vi "Main_16b.vi"() -> ()   [LabVIEW 2023]
uses:
  ENUM_Type.ctl
  Cluster_Tracking point.ctl
  Cluster_Point.ctl
  ENUM_Direction_a2.ctl
  Map_Direction Next.ctl
panel:
  out "left":i32
  out "Answer 2":i32
  out "Array 2":cluster{"Track Point":T1[]}[](array[cluster])
  out "Array":T4[][](array[typedef])
  in  "Puzzle":string="\\.......................|..-.............../../.......|...............\\.\\.....|..../.............|............\n........................../....../..............................-............-.-..--.........-...........\\/...\n....\\............../...........-...-......|.............................\\...............-........-....|.......\n......\\....|................./.\\................/..................../.......................|..\\......-......\n.................../..................-./.................../.....-...................|......\\.......|\\...\\./.\n.....|........../....................\\../..\\.../.\\.......-.............\\...........\\......|.\\..-..........-...\n..../............/.....\\...................../..--\\........|......\\....-...|.-...../......-........../........\n..............\\.-............./........./....|\\.......\\..........|.................|.|.................-......\n.....|..........-................-.../..........-........................\\.......|.........................-..\n.|.-......./....................\\........-.............../..\\.|.-\\...........\\./.................-............\n................|/............................../..-.\\..................-..../../...../.../..../..........|...\n........................./.....................\\..\\....-....../-.....................\\|.........././.-........\n...\\.....................-...../|............--......-..|...../.....|......|.../.\\....|.............\\|.......\\\n.........-...-.....|.........../...-/........|......./|............-.......-.....\\.............\\|....../......\n.....|...|.................|...../.............|.................../..........\\|..\\......|..|....-............\n...........................-.........\\......\\.............\\...................-.....-.\\.......-.....|.........\n.................-.............-......./.............-..\\./......|....-..-..........-....-............\\.......\n.\\..\\.......-......|........................\\.............-.......................|.........|\\.|..\\......--/..\n..........-.....||--........|........-....../...........|../...-.........../.....-.\\..........|.......-.......\n..........\\..........|..................\\.................-..../............/..........|.......-........../...\n..--......../..........-..|........./.........-...../........-.................|..\\............../.....-......\n.....\\.............|...../......../............./||..........................\\............|...................\n..-.................-|..-....................\\.................|...\\.....\\............./......-.......\\.......\n............-../......\\...../.-....-.....-....-./../......\\..|..|............................|.../..|.........\n-................./................................................|...............|....|.....-.....|....../..\n...........-...................|...........\\.......-..\\.......-...........|..-....../........|...............|\n.........|...|-........../...-..........|.........\\.....||......./....|...............\\......-......\\...../...\n....|.........|............\\.-.......................................-.......................|.-..|.\\...\\.-...\n.|....|....-/....................\\\\..........................|........\\|...|..............\\..|......-.\\../....\n..|.\\......|..../.....|.......-....................|.\\..\\............/......................|.....\\../../.....\n.......|\\\\.\\/......................./.............|................../.........|.....\\-.......................\n......................................../.../................\\-..............-................./......\\.......\n............../............/\\......./........................./......|............\\/..........................\n......./................|......../.........-............\\.../.|....../....|...../..../......../...............\n...................|............-\\........../...\\.......\\....\\.....-.........-./....|.........................\n.....-..-\\.................|\\...........................|..........\\........-...|.............................\n..............................-.............-.......\\......................../.......\\|.......|...-....-......\n\\...................\\..../.................\\................|......-...-............./.-......................\n........................./.|./...|..\\.-............|.-.....-..........\\....-..../.....|.......|...............\n.................../......../..................|.|...............|.......|\\.....|......|...............\\/..|..\n.........|....-......../........-./..|.../..|./...................-........|..................................\n..|../............-......-.........................-..|....-................-..\\....../...........|...........\n....................-...............|.../.....|..../......../...|.......\\.....-.....\\..............-..\\.-.....\n...........\\.........../............................................\\......-................-.......|.....-...\n..-............./.......-\\...........|-..-../............../................................../...............\n.................\\.......\\............../.|.......-...\\............................................\\.-........\n.\\....|....\\......|........./.....--......................................|................\\..|-..............\n......../...............-..........................|...........................-.............-\\.-..|..........\n.......|......|/...\\........./......../.....\\.........\\.......................-...........\\..\\................\n.-..-../.............|................./../.................\\........-......|.\\.....||...................\\|...\n/......../....\\.....|-..........\\..............-.....|............/\\......\\...//....................\\...-/....\n................-...........-.-\\-..........\\.-./......../-................./../.\\........................./...\n-.........-.....|.....-..|..|.........|...................-..........\\/.-.....................................\n......./...../......\\............-.|...............|..../.........|....\\.................../..............|...\n...........|.......|....|...............\\........................\\/..\\......................................\\.\n......\\........-.........................\\..........\\.............\\......................\\/.....\\..|..........\n......\\...........|.........../..-............./........................../...-......../...............\\..|...\n..|............\\../........../............\\...|.......................-...............\\-../.|...|\\.....\\......\n.|....\\.|....-|.........\\......./.................../.|........|....../.--.\\.....\\..............-\\\\.........-.\n......................./.......\\...........|.\\............-.....\\.............\\.........--......../.\\..-.|../.\n......../.............../......\\.\\....|.............../...........................-........-......../.........\n.......|\\.............|.../|/........../....\\.....-....|.............-......./........\\..\\........\\..|......-.\n.............../...........-.....\\..\\....-...../...|......\\...........................\\...|...........|/......\n.............|....../.................../..|.....................|.......|....//..............\\...............\n......./....\\............................-.........................-/......../|......-....|.............../...\n...........................|...................\\...............................-.................|...........\\\n.............................-......./..../...................\\.../...........-.|......................||.....\n\\....\\....\\...-./......../.........\\................./................\\...................|...........-.......\n................-.../............/\\..................\\.\\..-....../................./..........|...............\n......../...\\.......................\\.......\\..\\......|.....|../..........\\..........-.............|..........\n../.........................................-\\..........-.........|-./.....-...|..|.......\\........-...../../.\n.....|..........-......../|-..............|.................-...........|...\\.....................\\...........\n.......|..............\\....\\.....-............../..\\\\..\\.......-........./.........-..|...|................../\n..........-.......-.-................../.........\\\\...../.....|..........\\......./.|.............-...........\\\n..................................-..................|...........\\../\\...../..../...\\................/........\n...-.........................................................\\.|..............\\..................\\............\n-.|..|...................../../.|.......\\.....|.....\\.\\...\\.........-.................................../.....\n...\\./....../........\\.......-.................\\.........|............-.........../...........\\.|.........|.\\.\n..........-...\\.............-.-............-.-................/.....................|........|............-...\n|......./............/..|..............\\...............|.......|\\................/....|.........|.........\\..\\\n.....\\../\\./.....................-.............\\..................|.|.........................................\n............/......../.../.......\\............/.........................\\........................\\............\n....../..|.............../....................-.......\\................................................|.....\\\n................................../.......././.......\\.....|.\\......-.........-..||......../........-.//......\n........................\\.......|............-....-...../..............................-............-....|...-\n.....-.......|......\\..|.........-....|......\\......../..../.......\\..........|....\\.............||..\\........\n..........|...........-|.......\\.......-....../...../..........||.......................\\............-..|.....\n.................../../..............................|....|................/........|-....|................/..\n.....................\\................/............................/-........./...|.............\\...|..|\\.....\n.....\\..\\..........\\......../......|.........-....-..-..|...........\\....|./....\\.\\..\\............../.........\n.......-...............-....../...........-.......................|../...............|...|.........../..../...\n.............|.../..................\\..\\..........-........||................\\/...........-|..................\n.............-..............-\\.../.................|......\\...../..........\\...-.....-....../................\\\n.....-....................................-.........\\/............../.............................|...........\n./.|../......\\\\..........................................|..............\\|/..-\\..........................\\....\n...........-.........\\............./....-........-....-....-.........\\..\\....-\\...-...............--.........-\n..\\.............................\\............................./\\..........-.............-...-./........../....\n.................../........\\....|..-....|||./..............-......-./....................../..|...|..........\n......\\.........../............|\\...|.-................../....................|\\..|..\\.............-./......|.\n...........-...................-.|........................\\...............|/..-...\\...|/\\...........|.........\n............|..../..................................\\.......................\\........................-........\n.\\..........................|......|......../.|....................../.......\\......\\.............../.........\n..........-.../............/..........................|....-......................|.-................|.-......\n......../............-...|.....|......../-.....-|...|./.......-..................-\\...........................\n...............\\.\\/.-....././................-.../..../.............../-|.....-.......|......./..--...........\n..........-\\\\.|-................./../..|.-.....--................../.................../.|.......-............\n..\\.................-..............-...............\\.....|......................./..\\.....--........./..../..\\\n.......-....../..............|..................\\....|..|..........-.....|.|.-.........................\\......\n..../..\\...\\....................................||.|......................................|.......\\/.........-\n................\\-.-.....||....\\.........................-...................................................|"
  in  "Example":string=".|...\\....\n|.-.\\.....\n.....|-...\n........|.\n..........\n.........\\\n..../.\\\\..\n.-.-/..|..\n.|....-|.\\\n..//.|...."
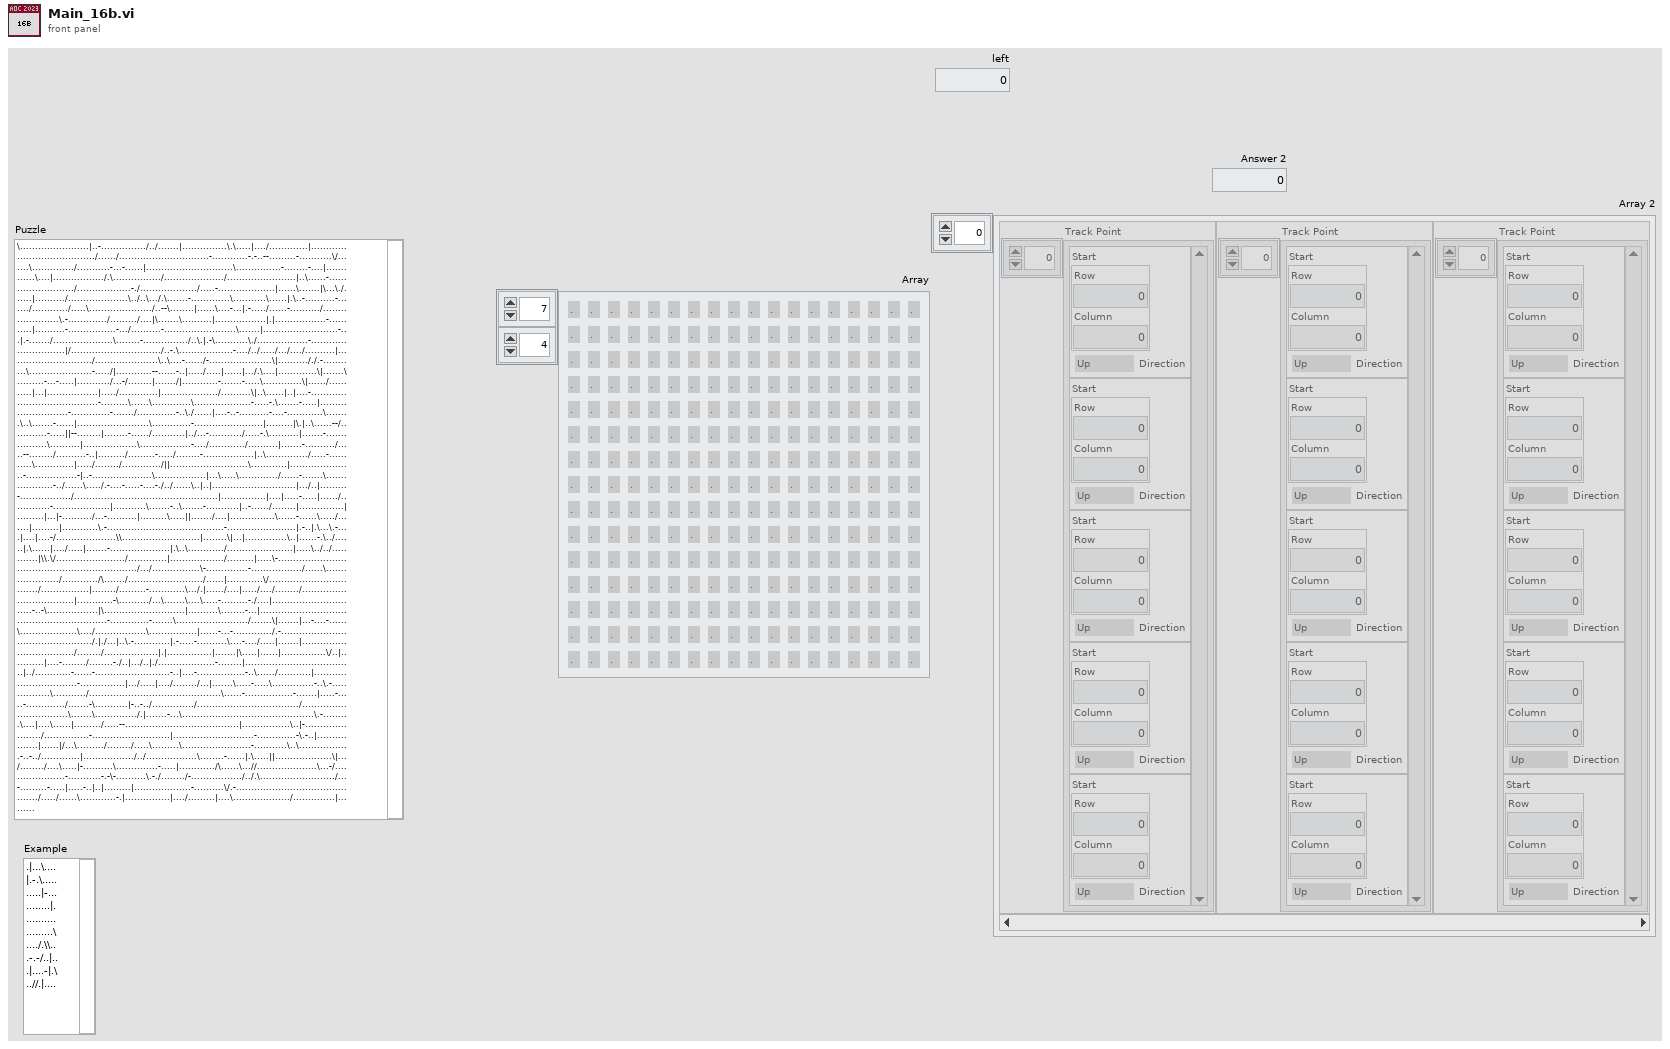
[diagram p1: front panel]
types:
  T1 = typedef "Cluster_Tracking point.ctl" = cluster{"Start":T2, "Direction":T3}
  T2 = typedef "Cluster_Point.ctl" = cluster{"Row":i32, "Column":i32}
  T3 = typedef "ENUM_Direction_a2.ctl" = enum16{"Up", "Left", "Down", "Right", "Up-Down", "Left-Right"}
  T4 = typedef "ENUM_Type.ctl" = enum16{".", "\\", "/", "|", "-"}
  T5 = typedef "Map_Direction Next.ctl" = map{T2, T3[]}
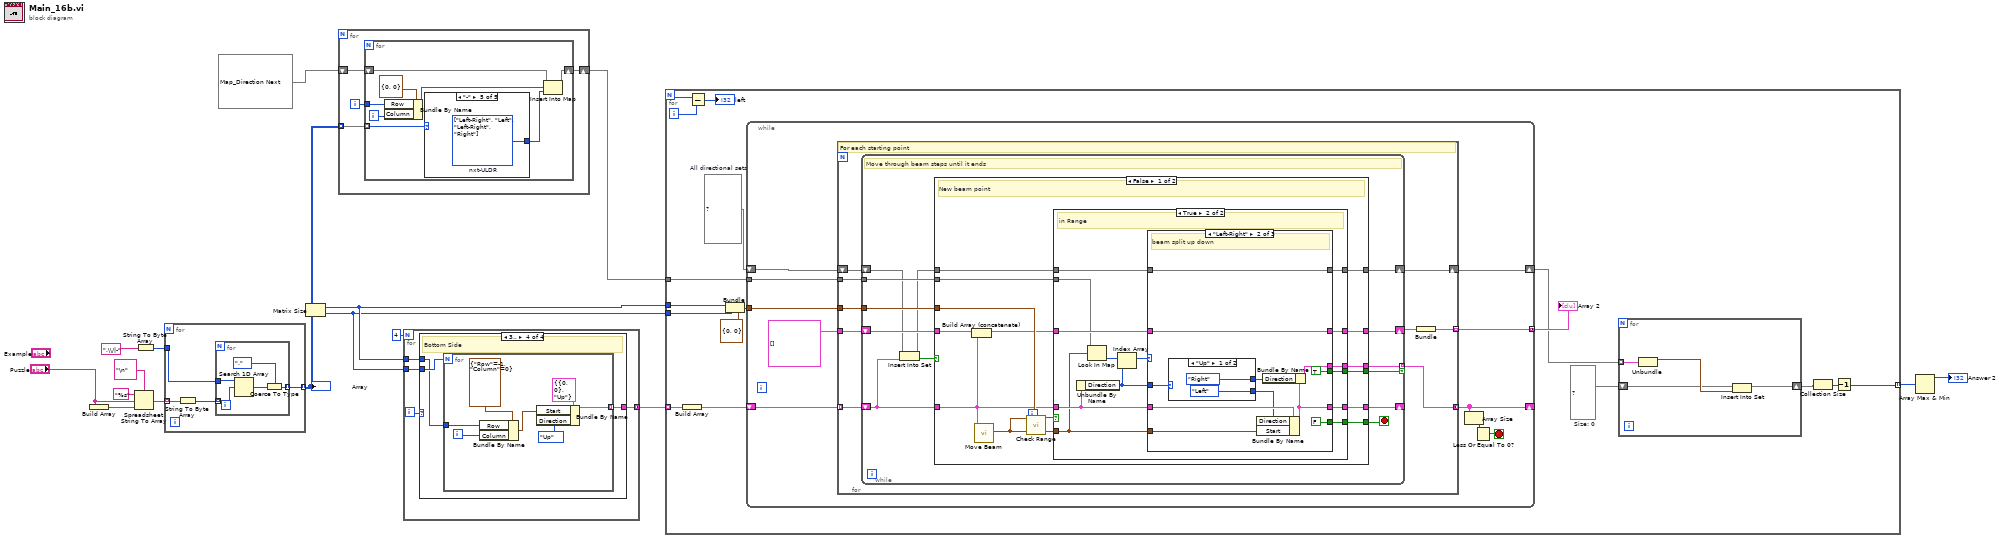
[diagram p0: block diagram]
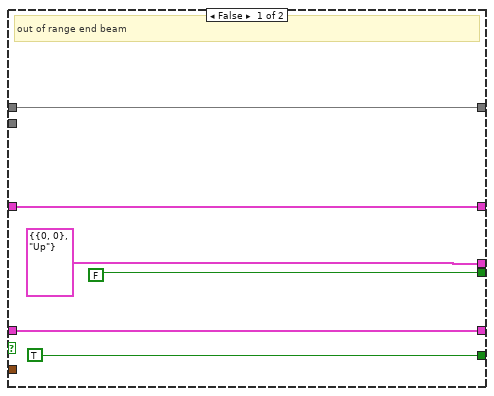
[diagram p2: hidden frame]
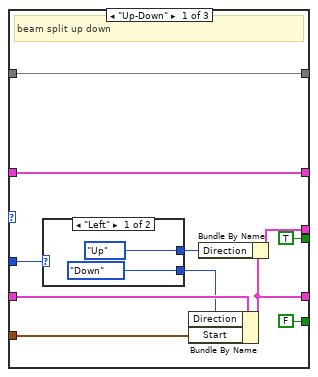
[diagram p3: hidden frame]
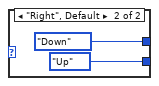
[diagram p4: hidden frame]
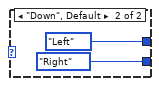
[diagram p5: hidden frame]
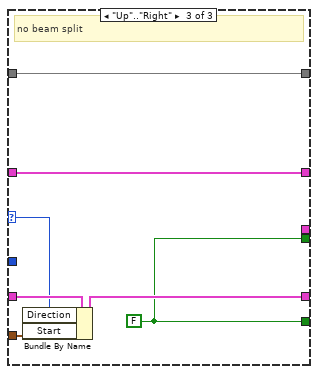
[diagram p6: hidden frame]
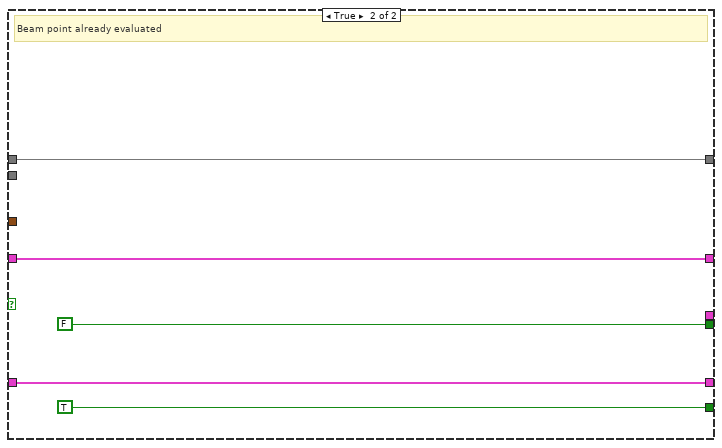
[diagram p7: hidden frame]
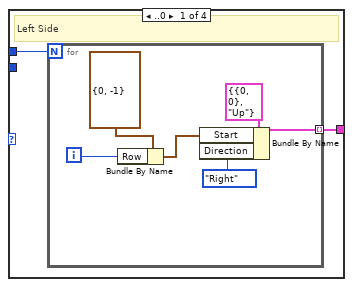
[diagram p8: hidden frame]
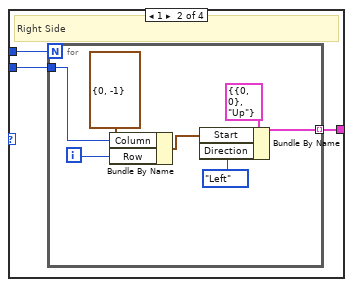
[diagram p9: hidden frame]
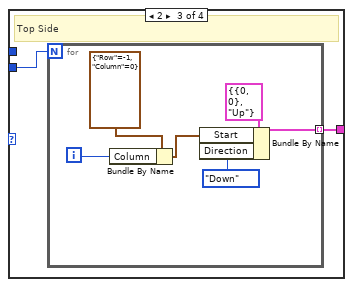
[diagram p10: hidden frame]
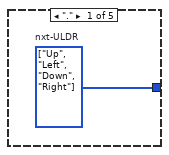
[diagram p11: hidden frame]
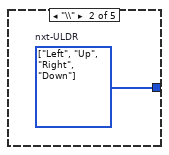
[diagram p12: hidden frame]
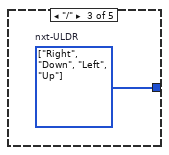
[diagram p13: hidden frame]
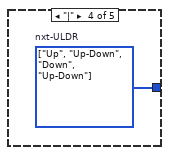
[diagram p14: hidden frame]
diagram:
  n1 = Build Array("Puzzle") -> (w16:string[])
  n2 = Spreadsheet String To Array(delimiter (Tab)="\n", format string="%s", spreadsheet string="Puzzle", array type (2D Dbl)=w16) -> (array=w13:string[])
  n3 = String To Byte Array(string=".\\/|-") -> (unsigned byte array=w11:u8[])
  n4 = for {
    tunnel: w13 -> [w20] mode=indexing
    tunnel: w11 -> [w19]
    tunnel: [w17] -> w10 mode=indexing
    n5 = String To Byte Array(string=w20) -> (unsigned byte array=w18:u8[])
    n6 = for {
      tunnel: w19 -> [w25]
      tunnel: w18 -> [w24] mode=indexing
      tunnel: [w21] -> w17 mode=indexing
      n7 = Search 1D Array(1D array=w25, element=w24) -> (index of element=w23:i32)  [unwired: 1 in]
      n8 = Coerce To Type(0:w23, 1:ENUM_Type."." ("Enum")) -> (2:w21:T4)
    }
  }
  "Array" <- w10
  n9 = Matrix Size(0:w10) -> (1:w4:i32, 2:w3:i32)
  n10 = for {
    tunnel: w10 -> [w29] mode=indexing
    shift-right: [w26] -> w8
    shift-left: T5 {} -> [w27]
    i -> [w28]
    n11 = for {
      tunnel: w29 -> [w37] mode=indexing
      tunnel: w28 -> [w35]
      shift-right: [w32] -> w26
      shift-left: w27 -> [w33]
      i -> [w34]
      n12 = Bundle By Name(cluster=T2 {"Row"=0, "Column"=0} ("Start"), "Row"=w35, "Column"=w34) -> (w31:T2)
      n13 = case shown="\"-\"" w37 {
        tunnel: [w38 w39 w40 w41 w42] -> w30
        frame "." {
          w38 = T3[] [enum."Up", enum."Left", enum."Down", enum."Right"] items=["Up", "Left", "Down", "Right", "Up-Down", "Left-Right"]  # nxt-ULDR
        }
        frame "\\" {
          w39 = T3[] [enum."Left", enum."Up", enum."Right", enum."Down"] items=["Up", "Left", "Down", "Right", "Up-Down", "Left-Right"]  # nxt-ULDR
        }
        frame "/" {
          w40 = T3[] [enum."Right", enum."Down", enum."Left", enum."Up"] items=["Up", "Left", "Down", "Right", "Up-Down", "Left-Right"]  # nxt-ULDR
        }
        frame "|" {
          w41 = T3[] [enum."Up", enum."Up-Down", enum."Down", enum."Up-Down"] items=["Up", "Left", "Down", "Right", "Up-Down", "Left-Right"]  # nxt-ULDR
        }
        frame "-" {
          w42 = T3[] [enum."Left-Right", enum."Left", enum."Left-Right", enum."Right"] items=["Up", "Left", "Down", "Right", "Up-Down", "Left-Right"]  # nxt-ULDR
        }
      }
      n14 = Insert Into Map(map in=w33, key=w31, value=w30) -> (map out=w32:T5)  [unwired: 2 out]
    }
  }
  n15 = for {
    N: 4 -> [_]
    tunnel: [w46] -> w6 mode=concatenating
    tunnel: w4 -> [w44]
    tunnel: w3 -> [w43]
    i -> [w45]
    n16 = case shown="3.." w45 {
      tunnel: [w48 w57 w66 w75] -> w46
      tunnel: w44 -> [w47 w56 _ w73]
      tunnel: w43 -> [_ w55 w65 w74]
      frame ..0 {
        # "Left Side"
        n17 = for {
          N: w47 -> [_]
          tunnel: [w53] -> w48 mode=indexing
          i -> [w49]
          n18 = Bundle By Name(cluster=T2 {"Row"=0, "Column"=-1} ("Point"), "Row"=w49) -> (w50:T2)
          n19 = Bundle By Name(cluster=T1 {"Start"={"Row"=0, "Column"=0}, "Direction"=enum."Up"} ("Track Point"), "Start"=w50, "Direction"=ENUM_Direction_a2."Right") -> (w53:T1)
        }
      }
      frame 1 {
        # "Right Side"
        n20 = for {
          N: w56 -> [_]
          tunnel: [w63] -> w57 mode=indexing
          tunnel: w55 -> [w58]
          i -> [w59]
          n21 = Bundle By Name(cluster=T2 {"Row"=0, "Column"=-1} ("Point"), "Column"=w58, "Row"=w59) -> (w60:T2)
          n22 = Bundle By Name(cluster=T1 {"Start"={"Row"=0, "Column"=0}, "Direction"=enum."Up"} ("Track Point"), "Start"=w60, "Direction"=ENUM_Direction_a2."Left") -> (w63:T1)
        }
      }
      frame 2 {
        # "Top Side"
        n23 = for {
          N: w65 -> [_]
          tunnel: [w71] -> w66 mode=indexing
          i -> [w67]
          n24 = Bundle By Name(cluster=T2 {"Row"=-1, "Column"=0} ("Point"), "Column"=w67) -> (w68:T2)
          n25 = Bundle By Name(cluster=T1 {"Start"={"Row"=0, "Column"=0}, "Direction"=enum."Up"} ("Track Point"), "Start"=w68, "Direction"=ENUM_Direction_a2."Down") -> (w71:T1)
        }
      }
      frame 3.. {
        # "Bottom Side"
        n26 = for {
          N: w74 -> [_]
          tunnel: [w81] -> w75 mode=indexing
          tunnel: w73 -> [w76]
          i -> [w77]
          n27 = Bundle By Name(cluster=T2 {"Row"=-1, "Column"=0} ("Point"), "Row"=w76, "Column"=w77) -> (w78:T2)
          n28 = Bundle By Name(cluster=T1 {"Start"={"Row"=0, "Column"=0}, "Direction"=enum."Up"} ("Track Point"), "Start"=w78, "Direction"=ENUM_Direction_a2."Up") -> (w81:T1)
        }
      }
    }
  }
  n29 = for {
    N -> [w85]
    tunnel: w8 -> [w99]
    tunnel: w4 -> [w98]
    tunnel: w3 -> [w97]
    tunnel: [w88] -> w2 mode=indexing
    tunnel: w6 -> [w87] mode=indexing
    i -> [w84]
    w92 = set{T2} {}  # Size: 0
    w94 = set{T1} {}  # All directional sets
    n30 = Build Array(w87) -> (w86:T1[])
    n31 = Subtract(x=w85, y=w84) -> (x-y=→"left":i32)
    n32 = Bundle(cluster=T2 {"Row"=0, "Column"=0} ("Point"), "Row"=w98, "Column"=w97) -> (w96:T2)
    n33 = while {
      tunnel: w99 -> [w113]
      shift-right: [w106] -> _
      shift-left: w86 -> [w111]
      shift-right: [w110] -> w89
      shift-left: w94 -> [w112]
      tunnel: w96 -> [w107]
      tunnel: [w104] -> w93 mode=concatenating
      stop <- w108 stop-if-true
      n34 = for {
        tunnel: w113 -> [w121]
        shift-right: [w122] -> w110
        shift-left: w112 -> [w118]
        tunnel: w111 -> [w117] mode=indexing
        tunnel: T1[] [] ("Track Point") -> [w119]
        tunnel: w107 -> [w120]
        tunnel: [w116] -> w106 mode=concatenating
        tunnel: [w114] -> w104 mode=indexing
        # "For each starting point"
        n35 = while {
          tunnel: w121 -> [w134]
          tunnel: w120 -> [w133]
          shift-right: [w135] -> w122
          shift-left: w118 -> [w125]
          shift-right: [w130] -> w115
          shift-left: w119 -> [w132]
          shift-right: [w127] -> _
          shift-left: w117 -> [w126]
          tunnel: [w129] -> w116 mode=indexing if=w128
          stop <- w131 stop-if-true
          # "Move through beam steps until it ends"
          n36 = Insert Into Set(10:w126, 11:w125) -> (2:w123:bool, 3:w124:set{T1})
          n37 = case shown="False" w123 {
            tunnel: [w149 w211] -> w135
            tunnel: w134 -> [w148 _]
            tunnel: w133 -> [w147 _]
            tunnel: w132 -> [w138 w207]
            tunnel: [w144 TRUE] -> w131
            tunnel: [w143 w207] -> w130
            tunnel: [w142 _] -> w129
            tunnel: [w141 FALSE] -> w128
            tunnel: [w140 w209] -> w127
            tunnel: w126 -> [w136 w209]
            tunnel: w124 -> [w139 w211]
            frame False {
              # "New beam point"
              n38 = Build Array (concatenate)(w138, w136) -> (w137:T1[])
              n39 = call "Move Beam.vi"("Track Point"=w136) -> ("Next Position Out"=w146:T2)  [unwired: 9 in, 1 out]
              n40 = call "Check Range.vi"("Range"=w147, "Next Position"=w146) -> ("In Range Out"=w145:bool)  [unwired: 9 in]
              n41 = case shown="True" w145 {
                tunnel: [w154 w169] -> w149
                tunnel: w136 -> [w150 w162]
                tunnel: w139 -> [w154 w168]
                tunnel: w137 -> [w151 w167]
                tunnel: w146 -> [_ w160]
                tunnel: w148 -> [_ w164]
                tunnel: [TRUE w159] -> w144
                tunnel: [w151 w165] -> w143
                tunnel: [T1 {"Start"={"Row"=0, "Column"=0}, "Direction"=enum."Up"} ("Track Point") w156] -> w142
                tunnel: [FALSE w158] -> w141
                tunnel: [w150 w166] -> w140
                frame False {
                  # "out of range end beam"
                }
                frame True {
                  # "in Range"
                  n42 = Unbundle By Name(w162) -> ("Direction"=w157:T3)
                  n43 = Look In Map(map=w164, key=w160) -> (value=w163:T3[])  [unwired: 1 in, 1 out]
                  n44 = Index Array(array=w163, index=w157) -> (element=w161:T3)
                  n45 = case shown="\"Left-Right\"" w161 {
                    selector: w161 -> [_ _ w200]
                    tunnel: w167 -> [w178 w193 w206]
                    tunnel: [w178 w193 w206] -> w165
                    tunnel: w168 -> [w179 w194 w205]
                    tunnel: [w179 w194 w205] -> w169
                    tunnel: w162 -> [w180 w195 w203]
                    tunnel: [w171 w186 w204] -> w166
                    tunnel: w160 -> [w174 w189 w202]
                    tunnel: [FALSE FALSE w201] -> w159
                    tunnel: [TRUE TRUE w201] -> w158
                    tunnel: w157 -> [w177 w192 _]
                    tunnel: [w173 w188 _] -> w156
                    frame "Up-Down" {
                      # "beam split up down"
                      n46 = case shown="\"Left\"" w177 {
                        tunnel: [ENUM_Direction_a2."Down" ("Direction") ENUM_Direction_a2."Up" ("Direction")] -> w176
                        tunnel: [ENUM_Direction_a2."Up" ("Direction") ENUM_Direction_a2."Down" ("Direction")] -> w175
                        frame "Left" {
                        }
                        frame "Right", Default {
                        }
                      }
                      n47 = Bundle By Name(cluster=w180, "Direction"=w176, "Start"=w174) -> (w171:T1)
                      n48 = Bundle By Name(cluster=w171, "Direction"=w175) -> (w173:T1)
                    }
                    frame "Left-Right" {
                      # "beam split up down"
                      n49 = case shown="\"Up\"" w192 {
                        tunnel: [ENUM_Direction_a2."Left" ("Direction") ENUM_Direction_a2."Right" ("Direction")] -> w191
                        tunnel: [ENUM_Direction_a2."Right" ("Direction") ENUM_Direction_a2."Left" ("Direction")] -> w190
                        frame "Up" {
                        }
                        frame "Down", Default {
                        }
                      }
                      n50 = Bundle By Name(cluster=w195, "Direction"=w191, "Start"=w189) -> (w186:T1)
                      n51 = Bundle By Name(cluster=w186, "Direction"=w190) -> (w188:T1)
                    }
                    frame "Up".."Right" {
                      w201 = FALSE
                      # "no beam split"
                      n52 = Bundle By Name(cluster=w203, "Direction"=w200, "Start"=w202) -> (w204:T1)
                    }
                  }
                }
              }
            }
            frame True {
              # "Beam point already evaluated"
            }
          }
        }
        n53 = Bundle("Track Point"=w115) -> (w114:cluster{"Track Point":T1[]})  [unwired: 1 in]
      }
      n54 = Array Size(array=w106) -> (size(s)=w109:i32)
      n55 = Less Or Equal To 0?(x=w109) -> (x <= 0?=w108:bool)
    }
    "Array 2" <- w93
    n56 = for {
      tunnel: w89 -> [w103] mode=indexing
      shift-right: [w100] -> w91
      shift-left: w92 -> [w101]
      n57 = Unbundle(w103) -> ("Start"=w102:T2)  [unwired: 1 out]
      n58 = Insert Into Set(10:w102, 11:w101) -> (3:w100:set{T2})  [unwired: 1 out]
    }
    n59 = Collection Size(1:w91) -> (0:w90:i32)
    n60 = Decrement(x=w90) -> (x-1=w88:i32)
  }
  n61 = Array Max & Min(array=w2) -> (max value=→"Answer 2":i32)  [unwired: 3 out]
